vi "Array-Reorder (DBL).vi"(3 "Index":i32[](array[numeric]), 4 "X":dbl[](array[numeric])) -> (1 "Reordered X":dbl[](array[numeric]))   [LabVIEW 2020]
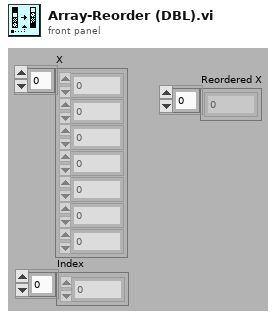
[diagram p1: front panel]
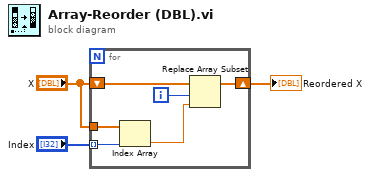
[diagram p0: block diagram]
diagram:
  n1 = for {
    tunnel: "X" -> [w8]
    tunnel: "Index" -> [w9] mode=indexing
    shift-right: [w4] -> w3
    shift-left: "X" -> [w7]
    i -> [w6]
    n2 = Index Array(array=w8, index=w9) -> (element=w5:dbl)
    n3 = Replace Array Subset(array=w7, new element=w5, index=w6) -> (w4:dbl[])
  }
  "Reordered X" <- w3
